vi "Test.vi"() -> ()   [LabVIEW 2020]
uses:
  Test typdef.ctl
  Write Section Path.vi
  Read Section Path.vi
  Generic Config Handling.lvlib
panel:
  in  "Section Name":string
  in  "Read":bool
  in  "Write":bool
  in  "stop":bool
  out "Output Data":T1
  out "Missing key(s)":bool
  out "Keys not found":string
  in  "Config Test":T1
  in  "configuration file path":path
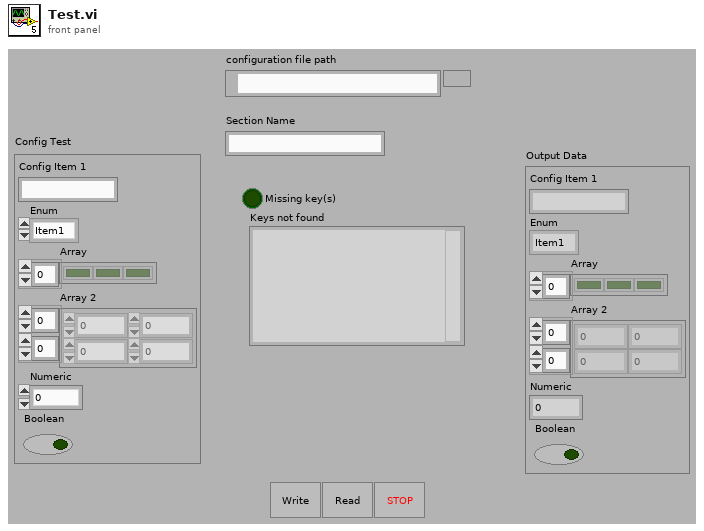
[diagram p1: front panel]
types:
  T1 = typedef "Test typdef.ctl" = cluster{"Config Item 1":string, "Enum":enum16{"Item1", "Item2", "Item3", "Item4"}, "Array":bool[], "Array 2":dbl[][], "Numeric":dbl, "Boolean":bool}
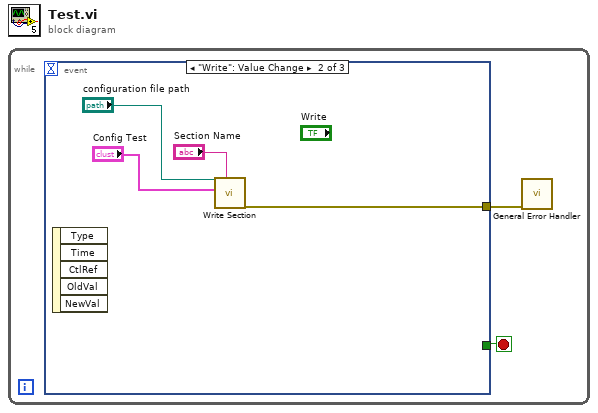
[diagram p0: block diagram]
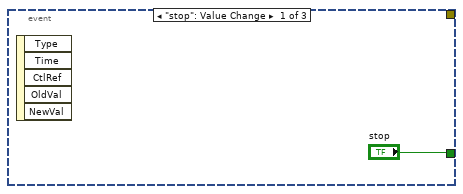
[diagram p2: hidden frame]
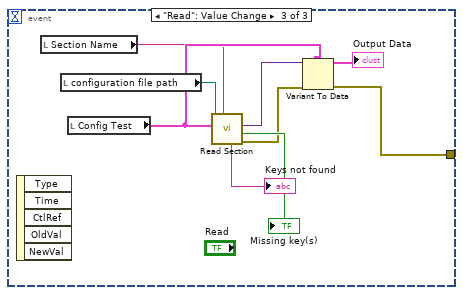
[diagram p3: hidden frame]
diagram:
  n1 = while {
    stop <- w2 stop-if-true
    n2 = event shown="[1] \"Write\": Value Change" {
      selector: _ -> [_ _ _]
      dyn-events: _ -> [_ _ _]
      timeout: _ -> [_ _ _]
      tunnel: ["stop" _ _] -> w2
      tunnel: [_ w4 w16] -> w1
      event "stop": Value Change {
        n3 = event-data() -> ()  [unwired: 1 in, 5 out]
      }
      event "Write": Value Change {
        n4 = event-data() -> ()  [unwired: 1 in, 5 out]
        n5 = call-poly "Write Section.vi"("Section Name"="Section Name", "Section (Cluster)"="Config Test", "Path in"="configuration file path") -> ("error out"=w4:errorcluster)  [unwired: 6 in, 2 out]
      }
      event "Read": Value Change {
        n6 = event-data() -> ()  [unwired: 1 in, 5 out]
        n7 = local read "Section Name"() -> (w12:string)
        n8 = local read "configuration file path"() -> (w14:path)
        n9 = local read "Config Test"() -> (w13:T1)
        n10 = call-poly "Read Section.vi"("Section Name"=w12, "Section (Cluster)"=w13, "Path in"=w14) -> ("error out"=w9:errorcluster, "Missing key(s)"=→"Missing key(s)":bool, "Section (Cluster) out"=w8:variant, "Keys not found"=→"Keys not found":string)  [unwired: 4 in, 1 out]
        n11 = Variant To Data(error in=w9, type=w13, Variant=w8) -> (data=→"Output Data":T1, error out=w16:errorcluster)
      }
    }
    n12 = call <vilib>:"General Error Handler.vi"("error in (no error)"=w1) -> ()  [unwired: 10 in, 5 out]
  }
